vi "备份参数.vi"() -> (0 "仪器公式":T2(array[cluster]), 1 "量程参数":T3(array[cluster]), 2 "试剂容量参数":T4, 3 "外设参数":cluster{"仪器版本":T1, "error out":errorcluster}, 5 "备份结果":string)   [LabVIEW 2022 SP3, in "斯坦道通用流路CODmn.lvlib"]
uses:
  <vilib>/NI/Progress Bar/Progress Bar.lvlib
  <vilib>/Utility/config.llb/NI_LVConfig.lvlib
  <userlib>/_OpenG.lib/variantconfig/variantconfig.llb/openg_variant_configuration_file.lvlib
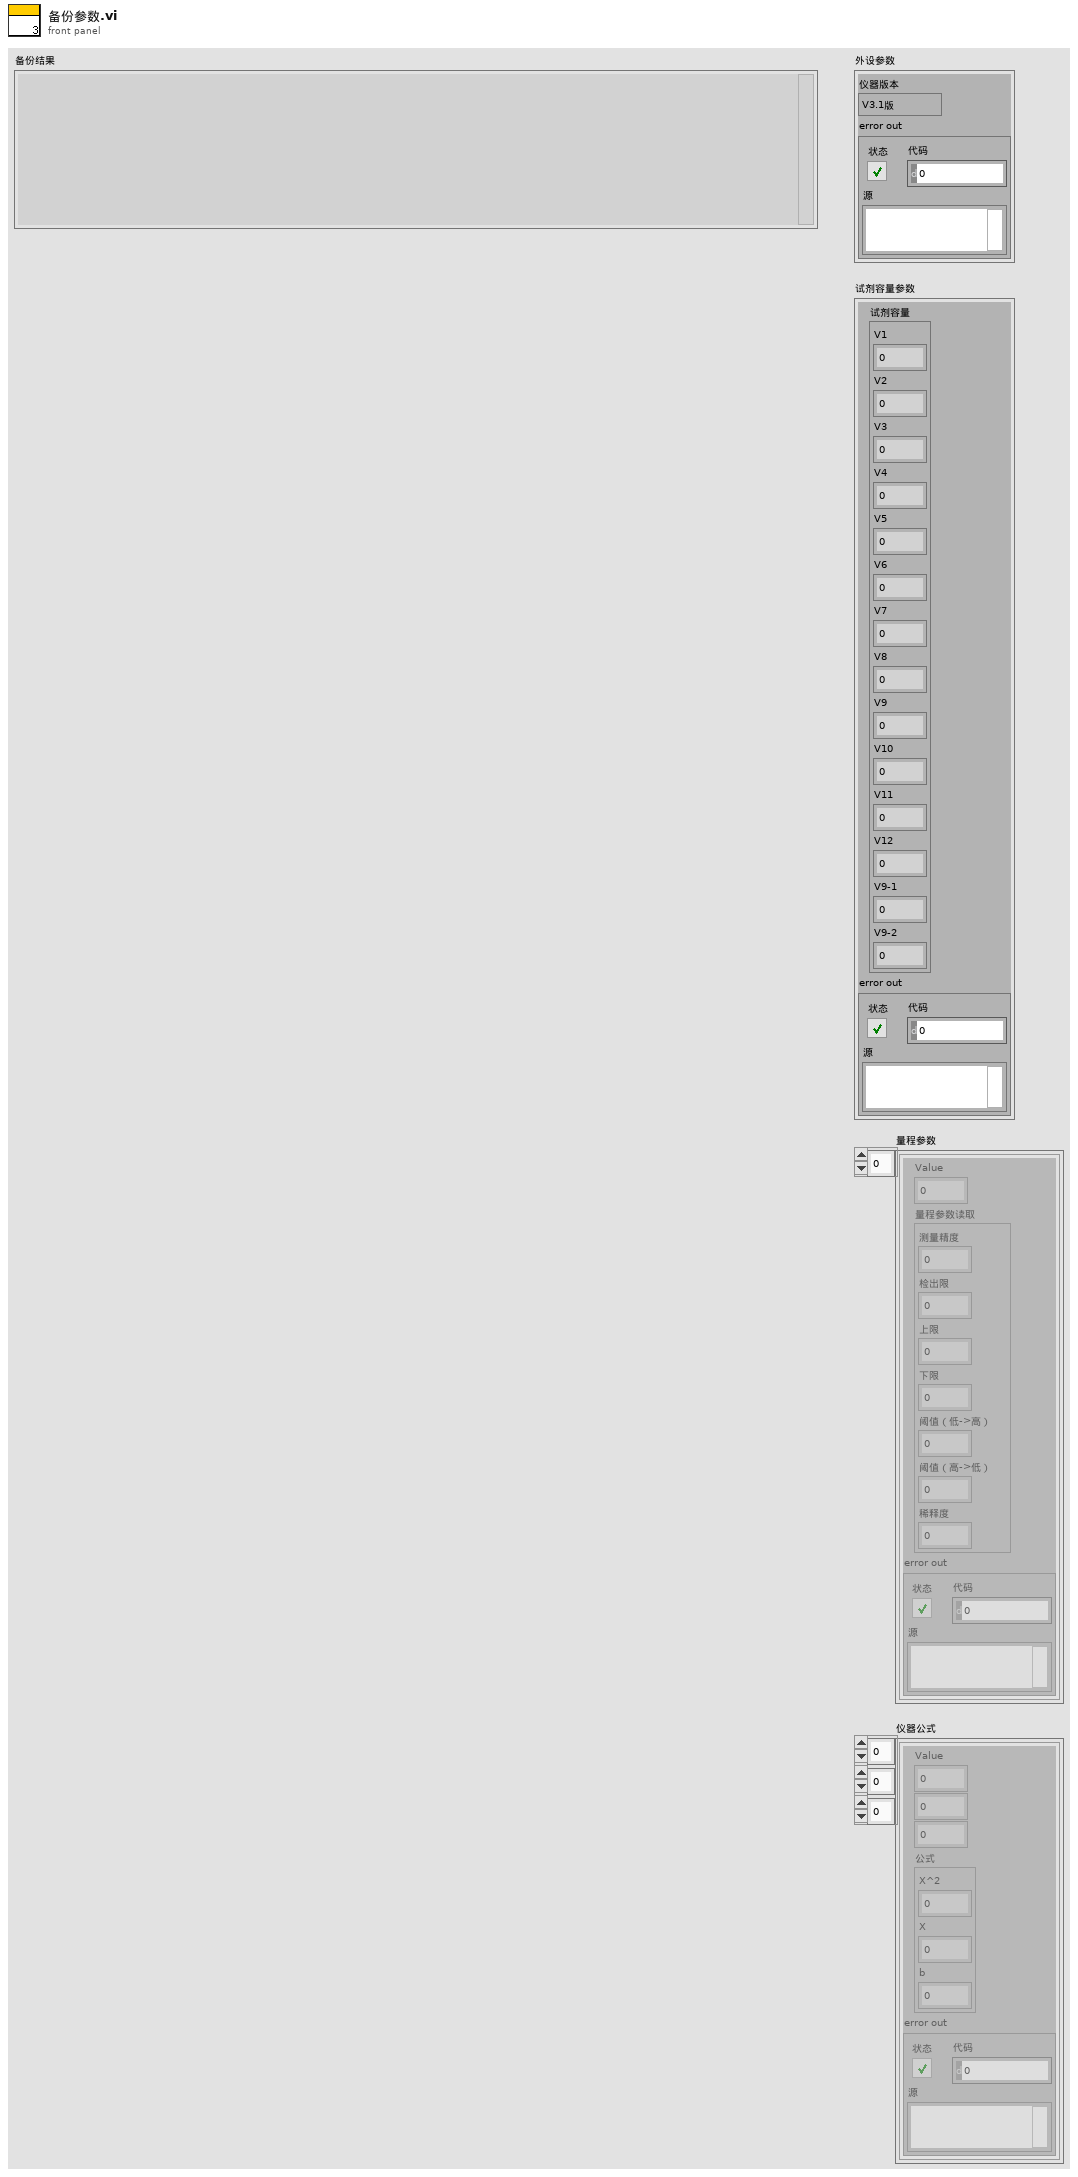
[diagram p1: front panel]
types:
  T1 = typedef "SingleStepTestV3.lvlib/SingleStepTestV3.lvclass/仪器版本.ctl" = enum16{"V3.1版", "V4版", "V3版", "V4.2版"}
  T2 = cluster{"Value":u16, i32, i32, "公式":cluster{"X^2":dbl, "X":dbl, "b":dbl}, "error out":errorcluster}[][][]
  T3 = cluster{"Value":u16, "量程参数读取":cluster{"测量精度":u16, "检出限":dbl, "上限":dbl, "下限":dbl, "阈值（低->高）":dbl, "阈值（高->低）":dbl, "稀释度":dbl}, "error out":errorcluster}[]
  T4 = cluster{"试剂容量":cluster{"V1":sgl, "V2":sgl, "V3":sgl, "V4":sgl, "V5":sgl, "V6":sgl, "V7":sgl, "V8":sgl, "V9":sgl, "V10":sgl, "V11":sgl, "V12":sgl, "V9-1":sgl, "V9-2":sgl}, "error out":errorcluster}
  T5 = enum16{"备份外设参数", "备份试剂容量参数", "备份量程参数", "备份仪器公式", "结束"}
  T6 = typedef "NI_LVConfig.lvlib/Config Data RefNum.ctl" = refnum<k1>
  T7 = typedef "斯坦道通用流路CODmn.lvlib/V3.1版外设参数.ctl" = cluster{"泵类型":u8, "进样速度":u32, "出样速度":u32, "泵阀量":u8, "阀方向":u8, "光谱仪类型":u8, "光谱采样次数":u8, "氙灯次数":u8, "B":u16, "C":u16, "D":u16, "E":u16, "B_COD":u16, "C_COD":u16, "D_COD":u16, "E_COD":u16, "G":u16, "M":u16, "N":u16, "氨氮注射泵控温下限":sgl, "氨氮注射泵控温上限":sgl, "总氮注射泵控温下限":sgl, "总氮注射泵控温上限":sgl, "消解温度下限":sgl, "消解温度上限":sgl, "加热10s限值":sgl, "KP":sgl, "KI":sgl, "KD":sgl, "高温高压阀开阀温度":sgl, "总氮x公式0":u8, "总氮x公式1":sgl, "总氮x公式2":sgl, "总磷浊度稀释系数":sgl, "总磷浊度补偿权重1":sgl, "总磷浊度补偿权重2":sgl, "盐度系数":sgl, "氨氮补偿系数1":sgl, "氨氮补偿系数2":sgl}
  T8 = typedef "斯坦道通用流路CODmn.lvlib/V4版外设参数.ctl" = cluster{"泵类型":u8, "注射泵正常速度":u32, "注射泵慢速":u32, "阀型号":u8, "res":u8, "光谱仪类型":u8, "光谱采样次数":u8, "氙灯次数":u8, "B":u16, "C":u16, "D":u16, "E":u16, "B_COD":u16, "C_COD":u16, "D_COD":u16, "E_COD":u16, "G":u16, "M":u16, "N":u16, "降温下限":sgl, "降温上限":sgl, "恒温温度下限":sgl, "恒温温度上限":sgl, "消解温度下限":sgl, "消解温度上限":sgl, "加热10s限值":sgl, "KP":sgl, "KI":sgl, "KD":sgl, "高温高压阀开阀温度":sgl, "总氮x公式0":u8, "总氮x公式1":sgl, "总氮x公式2":sgl, "总磷浊度稀释系数":sgl, "总磷浊度补偿权重1":sgl, "总磷浊度补偿权重2":sgl, "盐度系数":sgl, "氨氮补偿系数1":sgl, "氨氮补偿系数2":sgl, "缺试剂传感器阈值":u16}
  T9 = typedef "斯坦道通用流路CODmn.lvlib/V3版外设参数.ctl" = cluster{"泵类型":u8, "进样速度":u32, "出样速度":u32, "泵阀量":u8, "光谱仪类型":u8, "光谱采样次数":u8, "氙灯次数":u8, "B":u16, "C":u16, "D":u16, "E":u16, "B_COD":u16, "C_COD":u16, "D_COD":u16, "E_COD":u16, "G":u16, "M":u16, "N":u16, "氨氮注射泵控温下限":sgl, "氨氮注射泵控温上限":sgl, "总氮注射泵控温下限":sgl, "总氮注射泵控温上限":sgl, "消解温度下限":sgl, "消解温度上限":sgl, "加热10s限值":sgl, "高温高压阀开阀温度":sgl, "总氮x公式0":u8, "总氮x公式1":sgl, "总氮x公式2":sgl, "总磷浊度稀释系数":sgl, "总磷浊度补偿权重1":sgl, "总磷浊度补偿权重2":sgl, "盐度系数":sgl, "氨氮补偿系数1":sgl, "氨氮补偿系数2":sgl}
  T10 = typedef "斯坦道通用流路CODmn.lvlib/V4.2版外设参数.ctl" = cluster{"工作模式":u16, "泵类型":u16, "阀型号":u16, "注射泵进样速度":u16, "注射泵出样速度":u16, "注射泵滴定速度":u16, "res":u16, "注射泵慢速":u16, "光谱仪类型":u16, "光谱采样次数":u16, "氙灯次数":u16, "B":u16, "C":u16, "D":u16, "E":u16, "B_COD":u16, "C_COD":u16, "D_COD":u16, "E_COD":u16, "G":u16, "M":u16, "N":u16, "温度校准参数":sgl, "降温温度":sgl, "恒温温度":sgl, "消解温度":sgl, "高温高压阀开阀温度":sgl, "加热超时时间":sgl, "KP":sgl, "KI":sgl, "KD":sgl, "消解PID积分上限":sgl, "恒温PID积分上限":sgl, "PID积分下限":sgl, "缺试剂传感器阈值":u16, "滴定延时":u16, "滴定斜率阈值":sgl, "总氮x公式0":u16, "总氮x公式1":sgl, "总氮x公式2":sgl, "总磷浊度稀释系数":sgl, "总磷浊度补偿权重1":sgl, "总磷浊度补偿权重2":sgl, "盐度系数":sgl, "氨氮补偿系数1":sgl, "氨氮补偿系数2":sgl}
  T11 = cluster{"V1":sgl, "V2":sgl, "V3":sgl, "V4":sgl, "V5":sgl, "V6":sgl, "V7":sgl, "V8":sgl, "V9":sgl, "V10":sgl, "V11":sgl, "V12":sgl, "V9-1":sgl, "V9-2":sgl}
  T12 = cluster{"测量精度":u16, "检出限":dbl, "上限":dbl, "下限":dbl, "阈值（低->高）":dbl, "阈值（高->低）":dbl, "稀释度":dbl}
  T13 = cluster{"Value":u16, "量程参数读取":cluster{"测量精度":u16, "检出限":dbl, "上限":dbl, "下限":dbl, "阈值（低->高）":dbl, "阈值（高->低）":dbl, "稀释度":dbl}, "error out":errorcluster}
  T14 = cluster{"Value":u16, i32, i32, "公式":cluster{"X^2":dbl, "X":dbl, "b":dbl}, "error out":errorcluster}
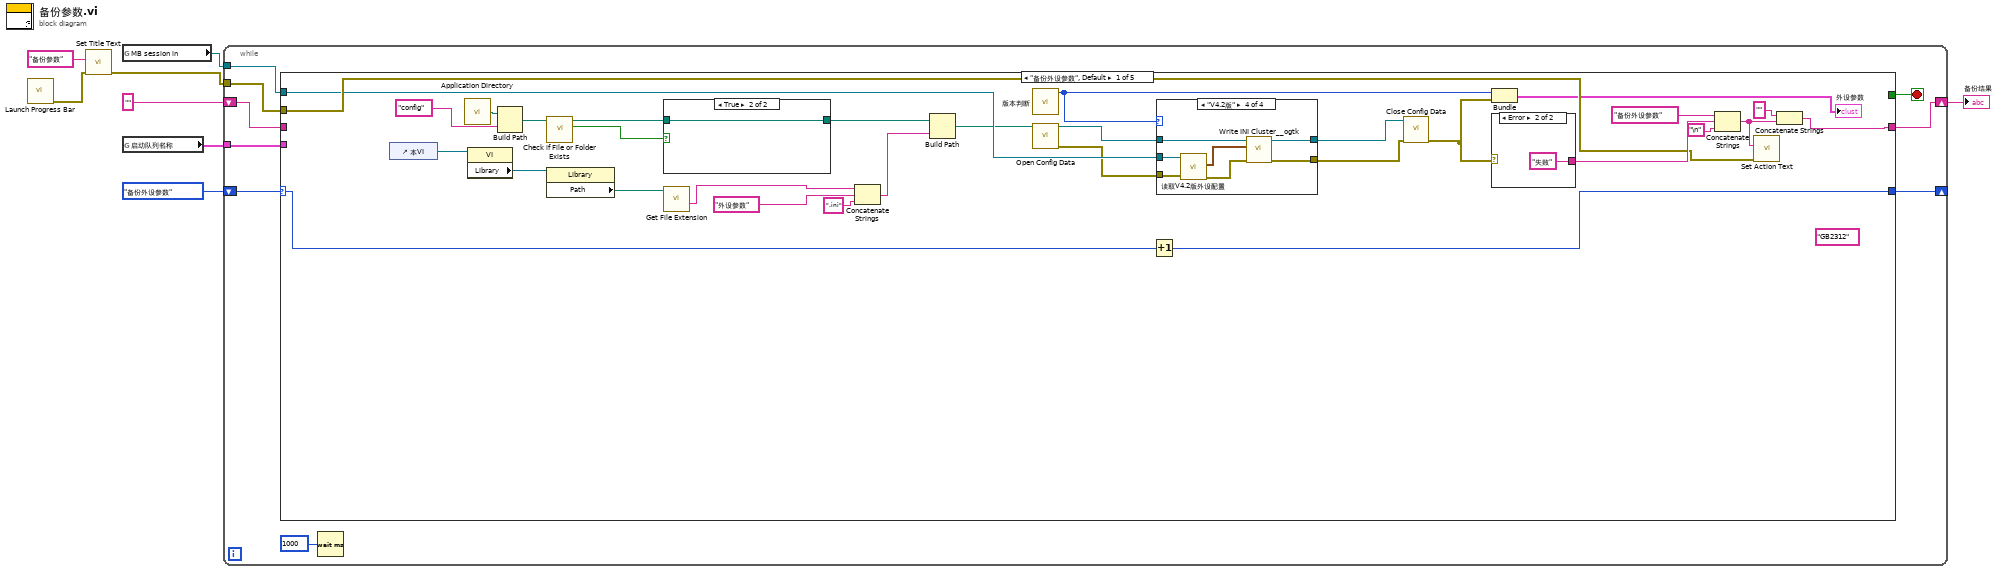
[diagram p0: block diagram]
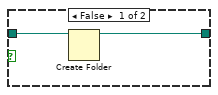
[diagram p2: hidden frame]
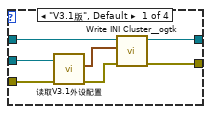
[diagram p3: hidden frame]
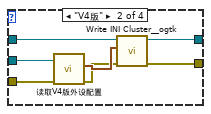
[diagram p4: hidden frame]
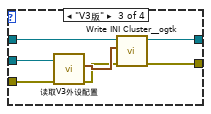
[diagram p5: hidden frame]
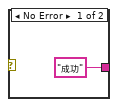
[diagram p6: hidden frame]
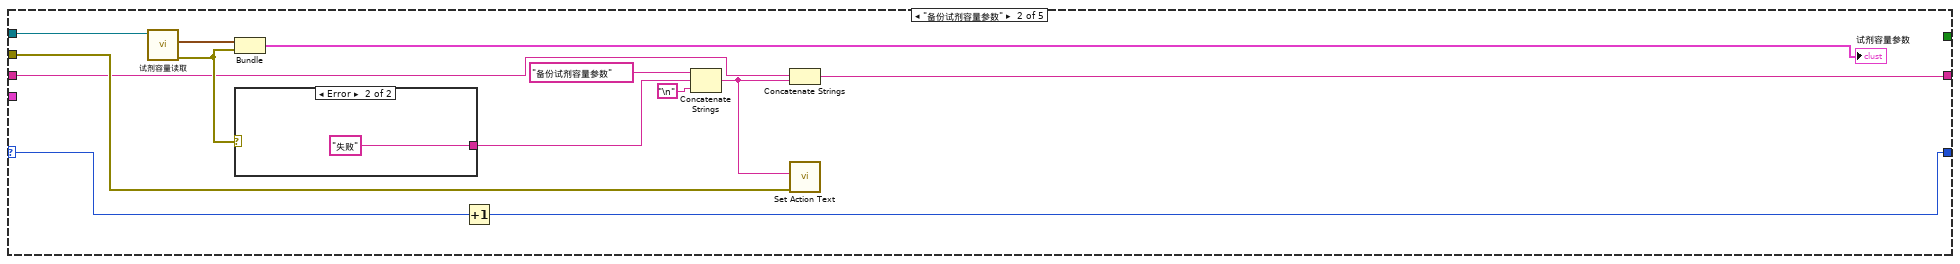
[diagram p7: hidden frame]
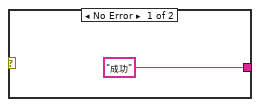
[diagram p8: hidden frame]
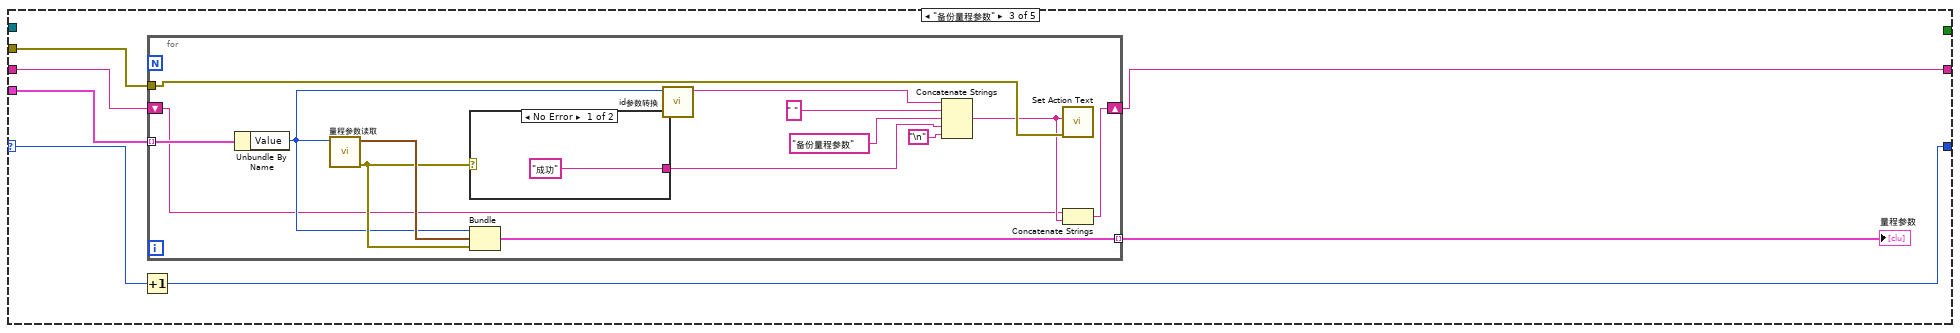
[diagram p9: hidden frame]
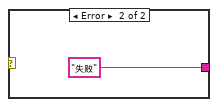
[diagram p10: hidden frame]
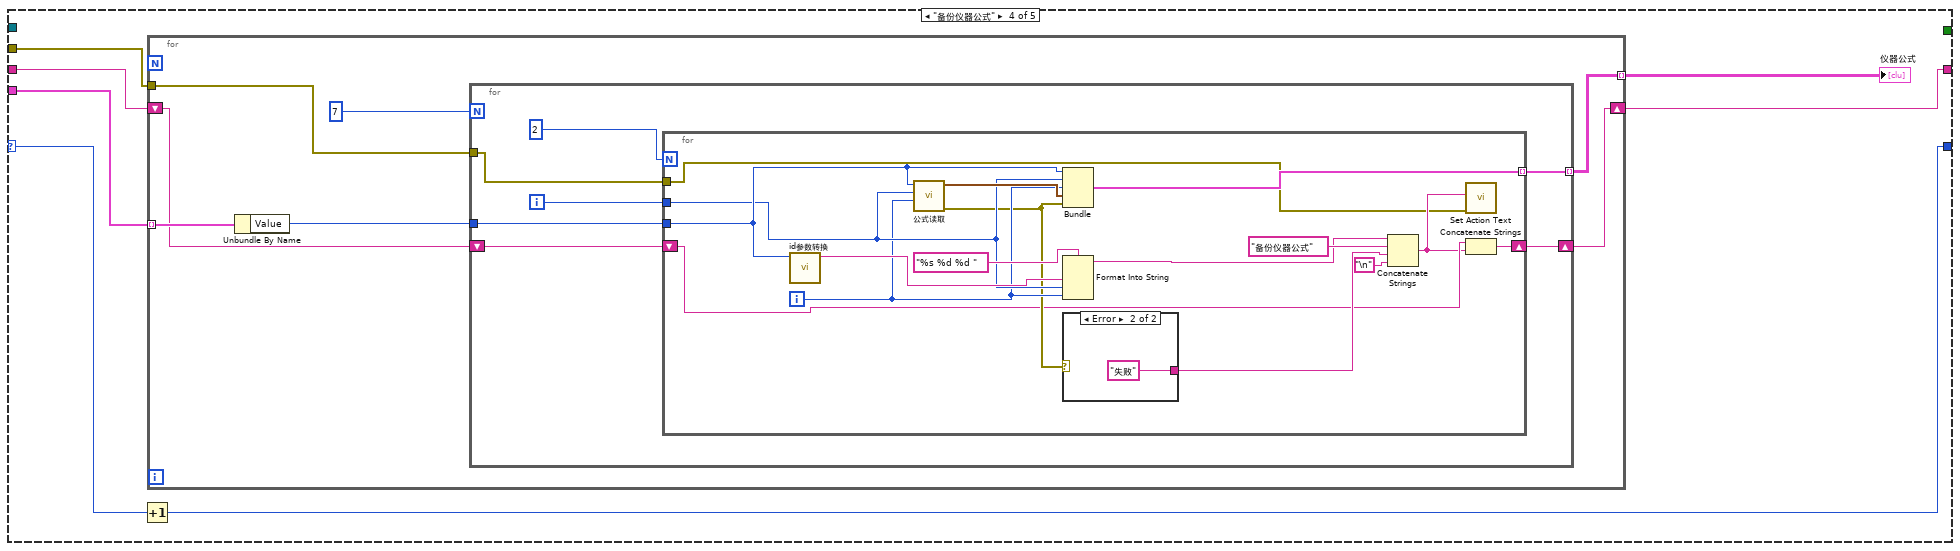
[diagram p11: hidden frame]
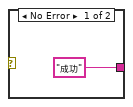
[diagram p12: hidden frame]
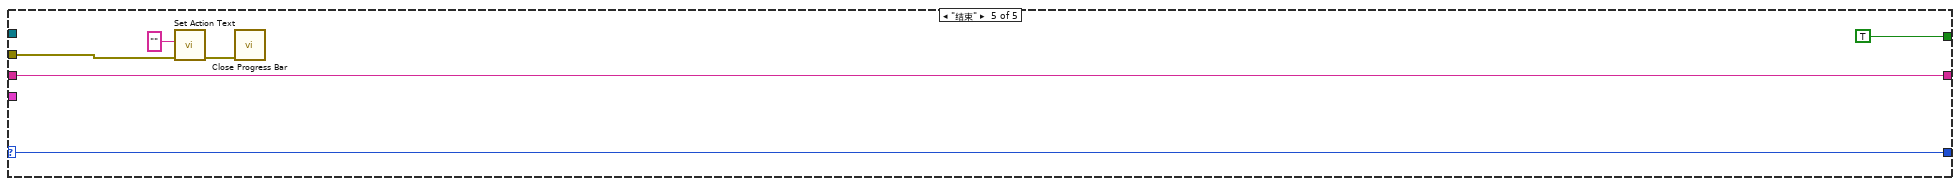
[diagram p13: hidden frame]
diagram:
  n1 = call <vilib>:"Launch Progress Bar.vi"() -> ("error out"=w3:errorcluster)  [unwired: 10 in, 1 out]
  n2 = call <vilib>:"Set Title Text.vi"("error in (no error)"=w3, "Installer Title"="备份参数") -> ("error out"=w2:errorcluster)  [unwired: 9 in]
  n3 = global read "VAR总磷总氮全局变量.vi" "MB session in"() -> (w7:refnum<class "MB_Master.lvclass">)
  n4 = global read "model config var.vi" "启动队列名称"() -> (w5:cluster{"String":string, "Value":u16}[])
  n5 = while {
    shift-right: [w13] -> _
    shift-left: T5."备份外设参数" ("枚举") -> [w16]
    tunnel: w7 -> [w17]
    shift-right: [w14] -> w4
    shift-left: "" -> [w15]
    tunnel: w5 -> [w12]
    tunnel: w2 -> [w10]
    stop <- w11 stop-if-true
    n6 = case shown="\"备份外设参数\", Default" w16 {
      selector: w16 -> [w45 w88 w100 w123 w164]
      tunnel: w17 -> [w39 w94 _ _ _]
      tunnel: w15 -> [_ w84 w102 w125 w163]
      tunnel: [w42 w82 w101 w124 w163] -> w14
      tunnel: [w44 w87 w99 w122 w164] -> w13
      tunnel: w12 -> [_ _ w103 w126 _]
      tunnel: [_ _ _ _ TRUE] -> w11
      tunnel: w10 -> [w40 w85 w97 w120 w161]
      frame "备份外设参数", Default {
        (unwired) "GB2312" ("XML Encoding")
        n7 = control-ref of="本VI"() -> (w25:refnum<vi>)
        n8 = call <vilib>:"Application Directory.vi"() -> ("Application Directory"=w35:path)
        n9 = property class="VI"(reference=w25) -> ("Library"=w37:refnum<vi>)  [unwired: 1 in, 2 out]
        n10 = Build Path(base path=w35, name or relative path="config" ("名称或相对路径")) -> (appended path=w33:path)
        n11 = call <vilib>:"Check if File or Folder Exists.vi"("path"=w33) -> ("file or folder exists?"=w30:bool, "dup path"=w29:path)  [unwired: 8 in, 1 out]
        n12 = property class="Library"(reference=w37) -> ("Path"=w36:path)  [unwired: 1 in, 2 out]
        n13 = case shown="True" w30 {
          tunnel: w29 -> [w50 w51]
          tunnel: [w49 w51] -> w28
          frame False {
            n14 = Create Folder(path (use dialog)=w50) -> (created path=w49:path)  [unwired: 2 in, 2 out]
          }
          frame True {
          }
        }
        n15 = call <vilib>:"Get File Extension.vi"("file"=w36) -> ("filename without extension"=w27:string)  [unwired: 6 in, 4 out]
        n16 = Concatenate Strings(w27, "外设参数" ("字符串"), ".ini" ("字符串")) -> (w31:string)
        n17 = Build Path(base path=w28, name or relative path=w31) -> (appended path=w23:path)
        n18 = call "版本判断.vi"() -> ("仪器版本"=w24:T1)  [unwired: 11 in]
        n19 = call <vilib>:"Open Config Data.vi"("configuration file path"=w23) -> ("error out"=w20:errorcluster, "refnum"=w22:T6)  [unwired: 8 in, 1 out]
        n20 = Increment(x=w45) -> (x+1=w44:T5)
        n21 = case shown="\"V4.2版\"" w24 {
          tunnel: [w52 w59 w66 w77] -> w19
          tunnel: w39 -> [w58 w65 w72 w76]
          tunnel: w22 -> [w54 w64 w71 w79]
          tunnel: [w53 w62 w69 w78] -> w21
          tunnel: w20 -> [w57 w61 w68 w75]
          frame "V3.1版", Default {
            n22 = call "读取V3.1外设配置.vi"("error in (no error)"=w57, "MB session in"=w58) -> ("error out"=w56:errorcluster, "外设配置"=w55:T7)  [unwired: 7 in, 1 out]
            n23 = call <userlib>:"Write INI Cluster__ogtk.vi"("error in (no error)"=w56, "INI Fomatted Cluster"=w55, "refnum"=w54) -> ("error out"=w52:errorcluster, "dup refnum"=w53:T6)  [unwired: 7 in]
          }
          frame "V4版" {
            n24 = call "读取V4版外设配置.vi"("error in (no error)"=w61, "MB session in"=w65) -> ("error out"=w60:errorcluster, "外设配置"=w63:T8)  [unwired: 7 in, 1 out]
            n25 = call <userlib>:"Write INI Cluster__ogtk.vi"("error in (no error)"=w60, "INI Fomatted Cluster"=w63, "refnum"=w64) -> ("error out"=w59:errorcluster, "dup refnum"=w62:T6)  [unwired: 7 in]
          }
          frame "V3版" {
            n26 = call "读取V3外设配置.vi"("error in (no error)"=w68, "MB session in"=w72) -> ("error out"=w67:errorcluster, "外设配置"=w70:T9)  [unwired: 7 in, 1 out]
            n27 = call <userlib>:"Write INI Cluster__ogtk.vi"("error in (no error)"=w67, "INI Fomatted Cluster"=w70, "refnum"=w71) -> ("error out"=w66:errorcluster, "dup refnum"=w69:T6)  [unwired: 7 in]
          }
          frame "V4.2版" {
            n28 = call "读取V4.2版外设配置.vi"("error in (no error)"=w75, "MB session in"=w76) -> ("error out"=w73:errorcluster, "外设配置"=w74:T10)  [unwired: 7 in, 1 out]
            n29 = call <userlib>:"Write INI Cluster__ogtk.vi"("error in (no error)"=w73, "INI Fomatted Cluster"=w74, "refnum"=w79) -> ("error out"=w77:errorcluster, "dup refnum"=w78:T6)  [unwired: 7 in]
          }
        }
        n30 = call <vilib>:"Close Config Data.vi"("error in (no error)"=w19, "refnum"=w21) -> ("error out"=w18:errorcluster)  [unwired: 8 in, 1 out]
        n31 = Bundle("仪器版本"=w24, "error out"=w18) -> (→"外设参数":cluster{"仪器版本":T1, "error out":errorcluster})  [unwired: 1 in]
        n32 = case shown="Error" w18 {
          tunnel: ["成功" "失败"] -> w48
          frame No Error {
          }
          frame Error {
          }
        }
        n33 = Concatenate Strings("备份外设参数" ("字符串"), w48, "\n") -> (w43:string)
        n34 = call <vilib>:"Set Action Text.vi"("error in (no error)"=w40, "Action Text"=w43) -> ()  [unwired: 9 in, 1 out]
        n35 = Concatenate Strings("" ("字符串"), w43) -> (w42:string)
      }
      frame "备份试剂容量参数" {
        n36 = call "试剂容量读取.vi"("MB session in"=w94) -> ("error out"=w89:errorcluster, "试剂容量"=w93:T11)  [unwired: 8 in, 1 out]
        n37 = Bundle("试剂容量"=w93, "error out"=w89) -> (→"试剂容量参数":T4)  [unwired: 1 in]
        n38 = case shown="Error" w89 {
          tunnel: ["成功" "失败"] -> w92
          frame No Error {
          }
          frame Error {
          }
        }
        n39 = Increment(x=w88) -> (x+1=w87:T5)
        n40 = Concatenate Strings("备份试剂容量参数" ("字符串"), w92, "\n") -> (w83:string)
        n41 = Concatenate Strings(w84, w83) -> (w82:string)
        n42 = call <vilib>:"Set Action Text.vi"("error in (no error)"=w85, "Action Text"=w83) -> ()  [unwired: 9 in, 1 out]
      }
      frame "备份量程参数" {
        n43 = Increment(x=w100) -> (x+1=w99:T5)
        n44 = for {
          tunnel: w103 -> [w117] mode=indexing
          tunnel: [w115] -> w98 mode=indexing
          shift-right: [w104] -> w101
          shift-left: w102 -> [w105]
          tunnel: w97 -> [w107]
          n45 = Unbundle By Name(w117) -> ("Value"=w111:u16)
          n46 = call "量程参数读取.vi"("测量参数"=w111) -> ("error out"=w112:errorcluster, "量程参数读取"=w116:T12)  [unwired: 9 in]
          n47 = case shown="No Error" w112 {
            tunnel: ["成功" "失败"] -> w114
            frame No Error {
            }
            frame Error {
            }
          }
          n48 = Bundle("Value"=w111, "量程参数读取"=w116, "error out"=w112) -> (w115:T13)  [unwired: 1 in]
          n49 = call "id参数转换.vi"("id"=w111) -> ("table输出"=w110:string)  [unwired: 9 in, 1 out]
          n50 = Concatenate Strings(w110, " " ("字符串"), "备份量程参数" ("字符串"), w114, "\n") -> (w106:string)
          n51 = call <vilib>:"Set Action Text.vi"("error in (no error)"=w107, "Action Text"=w106) -> ()  [unwired: 9 in, 1 out]
          n52 = Concatenate Strings(w105, w106) -> (w104:string)
        }
        "量程参数" <- w98
      }
      frame "备份仪器公式" {
        n53 = Increment(x=w123) -> (x+1=w122:T5)
        n54 = for {
          tunnel: w126 -> [w133] mode=indexing
          tunnel: [w130] -> w121 mode=indexing
          shift-right: [w128] -> w124
          shift-left: w125 -> [w129]
          tunnel: w120 -> [w127]
          n55 = Unbundle By Name(w133) -> ("Value"=w131:u16)
          n56 = for {
            N: 7 -> [_]
            tunnel: w131 -> [w140]
            tunnel: [w137] -> w130 mode=indexing
            shift-right: [w136] -> w128
            shift-left: w129 -> [w135]
            tunnel: w127 -> [w134]
            i -> [w139]
            n57 = for {
              N: 2 -> [_]
              tunnel: w140 -> [w152]
              tunnel: w139 -> [w149]
              tunnel: [w155] -> w137 mode=indexing
              shift-right: [w141] -> w136
              shift-left: w135 -> [w144]
              tunnel: w134 -> [w142]
              i -> [w148]
              n58 = call "id参数转换.vi"("id"=w152) -> ("table输出"=w150:string)  [unwired: 9 in, 1 out]
              n59 = call "公式读取.vi"("量程"=w148, "测量模式"=w149, "测量参数"=w152) -> ("error out"=w146:errorcluster, "公式"=w156:cluster{"X^2":dbl, "X":dbl, "b":dbl})  [unwired: 7 in]
              n60 = Bundle("Value"=w152, w149, w148, "公式"=w156, "error out"=w146) -> (w155:T14)  [unwired: 1 in]
              n61 = Format Into String(format string="%s %d %d " ("格式字符串"), w150, w149, w148) -> (resulting string=w147:string)  [unwired: 2 in, 1 out]
              n62 = case shown="Error" w146 {
                tunnel: ["成功" "失败"] -> w154
                frame No Error {
                }
                frame Error {
                }
              }
              n63 = Concatenate Strings(w147, "备份仪器公式" ("字符串"), w154, "\n") -> (w143:string)
              n64 = call <vilib>:"Set Action Text.vi"("error in (no error)"=w142, "Action Text"=w143) -> ()  [unwired: 9 in, 1 out]
              n65 = Concatenate Strings(w144, w143) -> (w141:string)
            }
          }
        }
        "仪器公式" <- w121
      }
      frame "结束" {
        n66 = call <vilib>:"Set Action Text.vi"("error in (no error)"=w161, "Action Text"="") -> ("error out"=w159:errorcluster)  [unwired: 9 in]
        n67 = call <vilib>:"Close Progress Bar.vi"("error in (no error)"=w159) -> ()  [unwired: 9 in, 2 out]
      }
    }
    n68 = Wait (ms)(milliseconds to wait=u32 1000 ("等待时间（毫秒）")) -> ()  [unwired: 1 out]
  }
  "备份结果" <- w4
